vi "DAQmx Read (Digital 1D Bool NChan 1Samp 1Line).vi"(0 "task/channels in":refnum<k21>, 9 "timeout":dbl=10.0 format="%0.2f", 11 "error in":errorcluster) -> (4 "task out":refnum<k21>, 6 "data":bool[](array[boolean]), 15 "error out":errorcluster)   [LabVIEW 2013]
doc: "Reads a single Boolean sample from each channel in a task that contains one or more digital input channels. Each channel must contain only a single digital line."
uses:
  nilvaiu.dll
panel:
  # "channel"
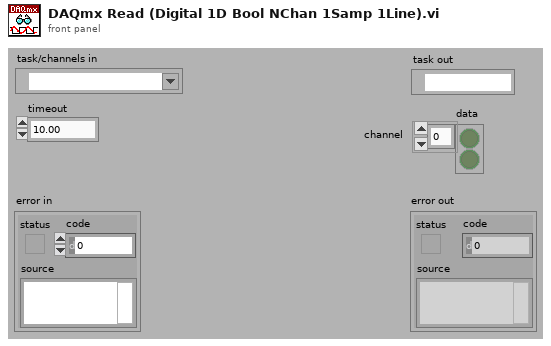
[diagram p1: front panel]
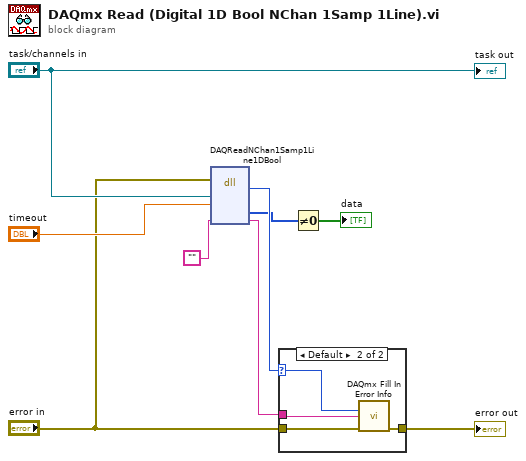
[diagram p0: block diagram]
diagram:
  n1 = dll-call lib="nilvaiu.*" fn="DAQReadNChan1Samp1Line1DBool"(error in="error in", "taskID"="task/channels in", "timeout"="timeout", "extendedErrorInfo"="") -> ("return type"=w7:i32, "data"=w3:u8[], "extendedErrorInfo"=w5:string)  [unwired: 4 in, 3 out]
  n2 = case shown="Default" w7 {
    selector: w7 -> [_ w13]
    tunnel: "error in" -> [w10 w14]
    tunnel: [w10 w12] -> w9
    tunnel: w5 -> [_ w11]
    frame 0 {
    }
    frame Default {
      n3 = call "DAQmx Fill In Error Info.vi"("status code"=w13, "extended error info"=w11, "error in"=w14) -> ("error out"=w12:errorcluster)  [unwired: 1 in, 11 out]
    }
  }
  "error out" <- w9
  n4 = Not Equal To 0?(x=w3) -> (x != 0?=→"data":bool[])
  "task out" <- "task/channels in"
